vi "Check-speed.vi"(8 "error in (no error)":errorcluster, 10 "Speed in":dbl, 11 "Motor-Serial in":refnum<class "Motor-Serial.lvclass">) -> (0 "error out":errorcluster, 1 "In range?":bool, 2 "Speed out":dbl, 3 "Motor-Serial out":refnum<class "Motor-Serial.lvclass">)   [LabVIEW 2013, in "PowderDeposition.lvlib" / "Motor-Serial.lvclass"]
uses:
  Motor-Serial.lvclass
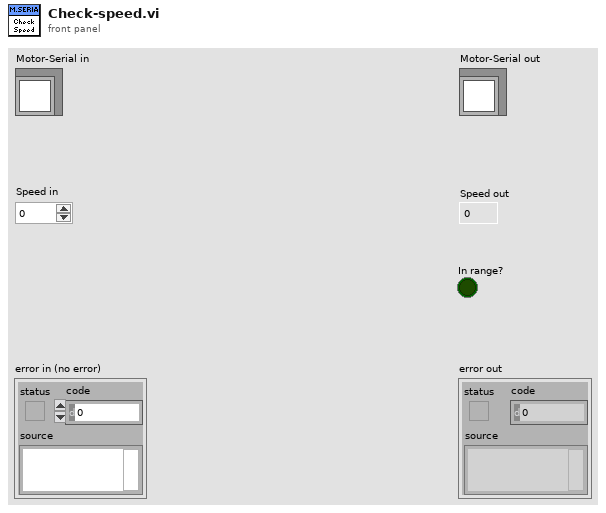
[diagram p1: front panel]
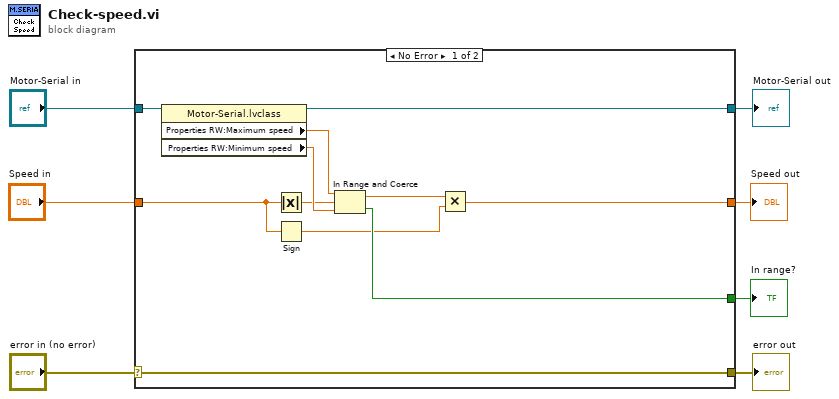
[diagram p0: block diagram]
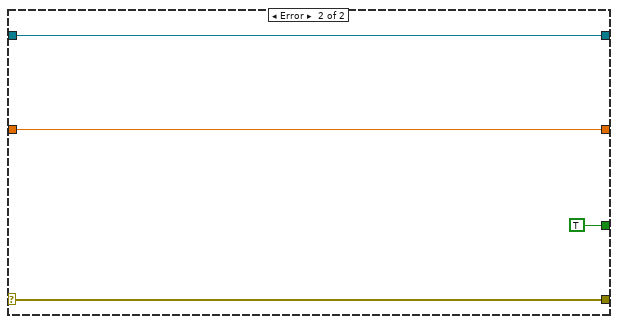
[diagram p2: hidden frame]
diagram:
  n1 = case shown="No Error" "error in (no error)" {
    selector: "error in (no error)" -> [w17 w22]
    tunnel: [w17 w22] -> w6
    tunnel: [w16 w21] -> w4
    tunnel: "Motor-Serial in" -> [w18 w21]
    tunnel: "Speed in" -> [w10 w19]
    tunnel: [w15 TRUE] -> w2
    tunnel: [w9 w19] -> w1
    frame No Error {
      n2 = property class="Motor-Serial.lvclass"(reference=w18) -> (reference out=w16:refnum<class "Motor-Serial.lvclass">, "Properties RW:Maximum speed"=w13:dbl, "Properties RW:Minimum speed"=w12:dbl)  [unwired: 1 in, 1 out]
      n3 = Absolute Value(x=w10) -> (abs(x)=w11:dbl)
      n4 = Sign(1:w10) -> (0:w8:dbl)
      n5 = In Range and Coerce(upper limit=w13, x=w11, lower limit=w12) -> (coerced(x)=w14:dbl, In Range?=w15:bool)
      n6 = Multiply(x=w14, y=w8) -> (x*y=w9:dbl)
    }
    frame Error {
    }
  }
  "error out" <- w6
  "Motor-Serial out" <- w4
  "Speed out" <- w1
  "In range?" <- w2
